vi "Change Sine Ramp Start.vi"(8 "error in":errorcluster, 10 "Start point":T1, 11 "TEC 1090 in":refnum<class "Meerstetter TEC.lvclass">) -> (0 "error out":errorcluster, 3 "TEC 1090 out":refnum<class "Meerstetter TEC.lvclass">)   [LabVIEW 2014, in "Meerstetter Lib.lvlib" / "Meerstetter TEC.lvclass"]
uses:
  Meerstetter TEC.lvclass
  Controls/Sine ramp start point.ctl
  reusable/Session APIs/Serial/Serial Session.lvclass
  Meerstetter TEC.lvclass/Meerstetter TEC.ctl
  Configurable Device/Configurable Device.lvclass/Configurable Device.ctl
  Accessors/Read SerialSession.vi
  Configurable Device/Read Log Session.vi
  Configurable Device/Read ID.vi
  reusable/Session APIs/Serial/Public/Asynchronous Write.vi
  reusable/Session APIs/Serial/Public/Asynchronous Read.vi
  <userlib>/_Session Fwk/Session - Root.lvclass
  reusable/Session APIs/Session Log/System Log.lvclass
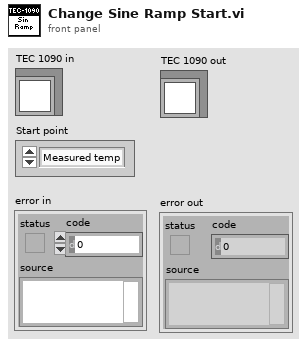
[diagram p1: front panel]
types:
  T1 = typedef "Sine ramp start point.ctl" = enum16{"Measured temp", "Target temp"}
  T2 = typedef "Session - Root.lvclass/Session Handle.ctl" = refnum<data-value>
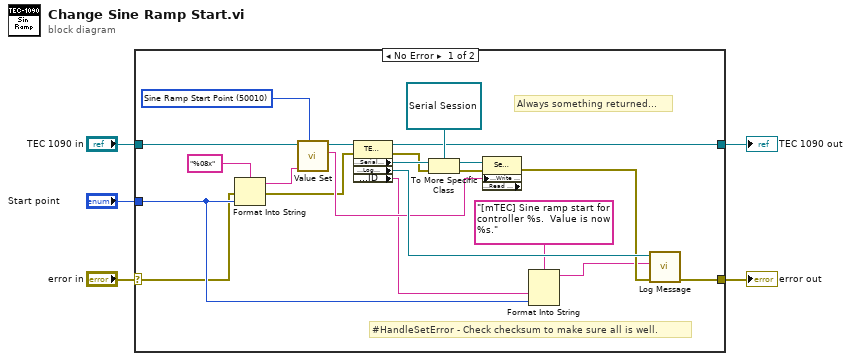
[diagram p0: block diagram]
diagram:
  n1 = case shown="No Error" "error in" {
    selector: "error in" -> [w10 w28]
    tunnel: [w18 w28] -> w4
    tunnel: [w20 w27] -> w2
    tunnel: "TEC 1090 in" -> [w26 w27]
    tunnel: "Start point" -> [w12 _]
    frame No Error {
      w6 = u16 50010 items=["Input Selection"=2000, "Status"=2010, "Set Current"=2020, "Set Voltage"=2021, "Current Limitation"=2030, "Voltage Limitation"=2031, "Current Error Threshold"=2032, "Voltage Error Threshold"=2033, "Channel Baud Rate"=2050, "Response Delay"=2052, "Timeout"=2060, "Target Object Temperature"=3000, "Proximity Width"=3002, "Coarse Temp Ramp"=3003, "Kp"=3010, "Ti"=3011, "Td"=3012, "D Part Damping D1"=3013, "Live Enable"=50000, "Live Set Current"=50001, "Live Set Voltage"=50002, "Sine Ramp Start Point"=50010, "Object Target Temp Source"=50011, "Object Target Temperature"=50012, "Save Data to Flash"=108] ("Value Set")
      # "Always something returned..."
      # "#HandleSetError - Check checksum to make sure all is well."
      n2 = Format Into String(format string="%08x", error in=w10, w12) -> (resulting string=w15:string, error out=w9:errorcluster)  [unwired: 1 in]
      n3 = call "Value Set.vi"("Value Set"=w6, "Value"=w15, "TEC 1090"=w26) -> ("hex integer string"=w13:string, "TEC 1091"=w25:refnum<class "Meerstetter TEC.lvclass">)  [unwired: 7 in]
      n4 = property class="TEC 1090"(reference=w25, error in=w9) -> (reference out=w20:refnum<class "Meerstetter TEC.lvclass">, error out=w8:errorcluster, "Accessors:SerialSession"=w24:T2, "Accessors:Log Session"=w19:T2, "Accessors:ID"=w7:string)
      n5 = To More Specific Class(target class=refnum<data-value> refnum, reference=w24, error in=w8) -> (specific class reference=w22:refnum<data-value>, error out=w21:errorcluster)
      n6 = property class="Serial Session" props=["Public:Write - Asynchronous", "Public:Read - Asynchronous"](reference=w22, error in=w21, "Public:Write - Asynchronous"=w13) -> (error out=w17:errorcluster)  [unwired: 2 out]
      n7 = Format Into String(format string="[mTEC] Sine ramp start for controller %s.  Value is now %s.", w7, w12) -> (resulting string=w11:string)  [unwired: 2 in, 1 out]
      n8 = call "Log Message.vi"("error in"=w17, "MSG In"=w11, "session in"=w19) -> ("error out"=w18:errorcluster)  [unwired: 7 in, 1 out]
    }
    frame Error {
    }
  }
  "error out" <- w4
  "TEC 1090 out" <- w2
